vi "readFromXML.vi"(8 "error in (no error)":errorcluster, 10 "XML in":string, 11 "TCSDebug in":refnum<class "TCSDebug.lvclass">) -> (0 "error out":errorcluster, 3 "TCSDebug out":refnum<class "TCSDebug.lvclass">)   [LabVIEW 2014, in "TCSDataDefinitions.lvlib" / "TCSCommand.lvlib" / "TCSDebug.lvclass"]
uses:
  TCSDebug.lvclass
  Enumerations/TCSDebuLevelTypes.ctl
  TCSDebug.lvclass/TCSDebug.ctl
  TCSTcsCommand/TCSTcsCommand.lvclass
  <userlib>/Common/XML/XMLParser/XMLParser.lvclass
  TCSCommand.lvlib
panel:
  out "debugLevel":T1
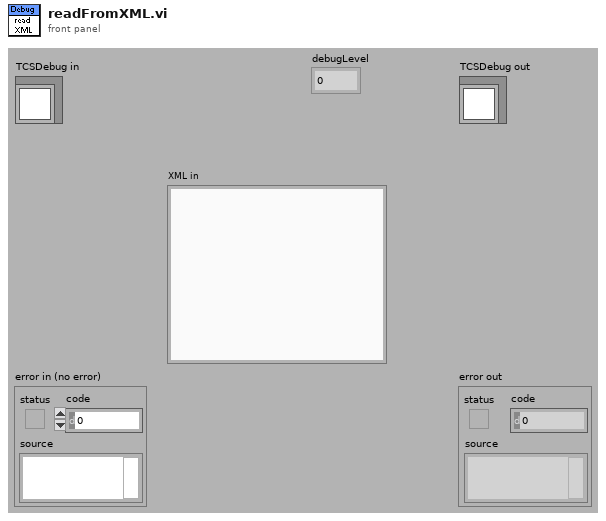
[diagram p1: front panel]
types:
  T1 = typedef "TCSDataDefinitions.lvlib/TCSCommand.lvlib/TCSDebuLevelTypes.ctl" = enum16{"0", "1", "2", "3", "4", "5", "6", "7", "8", "9", "10"}
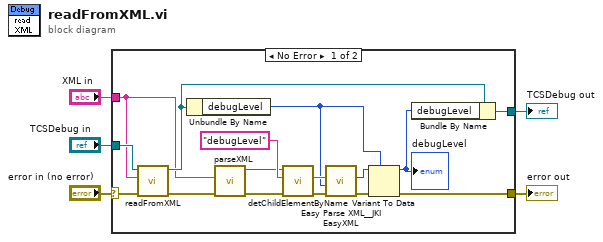
[diagram p0: block diagram]
diagram:
  n1 = case shown="No Error" "error in (no error)" {
    selector: "error in (no error)" -> [w16 w23]
    tunnel: [w8 w23] -> w4
    tunnel: [w19 w22] -> w2
    tunnel: "TCSDebug in" -> [w18 w22]
    tunnel: "XML in" -> [w14 _]
    frame No Error {
      n2 = call-parent "readFromXML.vi"("error in (no error)"=w16, "XMLin"=w14, "TCSTcsCommand in"=w18) -> ("error out"=w15:errorcluster, "TCSTcsCommand out"=w17:refnum<class "TCSDebug.lvclass">)  [unwired: 7 out]
      n3 = Unbundle By Name(w17) -> ("debugLevel"=w10:T1)
      n4 = call <userlib>:"parseXML.vi"("error in (no error)"=w15, "XMLString in"=w14) -> ("error out"=w20:errorcluster, "Element out"=w6:refnum<class "XMLParser.lvclass">)  [unwired: 8 in]
      n5 = call <userlib>:"detChildElementByName.vi"("error in (no error)"=w20, "childName"="debugLevel" ("ChildName"), "Element in"=w6) -> ("error out"=w7:errorcluster, "childXML"=w11:string)  [unwired: 5 in, 2 out]
      n6 = call <vilib>:"Easy Parse XML__JKI EasyXML.vi"("error in (no error)"=w7, "LabVIEW Data (Type)"=w10, "XML String"=w11) -> ("error out"=w13:errorcluster, "LabVIEW Data"=w12:variant)  [unwired: 7 in]
      n7 = Variant To Data(error in=w13, type=w10, Variant=w12) -> (data=w9:T1, error out=w8:errorcluster)
      "debugLevel" <- w9
      n8 = Bundle By Name(cluster=w17, "debugLevel"=w9) -> (w19:refnum<class "TCSDebug.lvclass">)
    }
    frame Error {
    }
  }
  "error out" <- w4
  "TCSDebug out" <- w2
